vi "Get JSON Data.vi"(7 "Panel Origin":T1, 8 "error in (no error)":errorcluster, 9 "Force Get All Data":bool, 10 "VI Reference":refnum<vi>, 11 "Boolean In":refnum<class "Boolean.lvclass">) -> (0 "error out":errorcluster, 2 "JSON string":string, 3 "Boolean Out":refnum<class "Boolean.lvclass">)   [LabVIEW 2015, in "Front Panel Publisher.lvlib" / "Boolean.lvclass"]
uses:
  Boolean.lvclass
  <vilib>/Utility/miscctls.llb/LVPointTypeDef.ctl
  Text_class/Text.lvclass
  Control_class/Control.lvclass
  Object_class/Object.lvclass
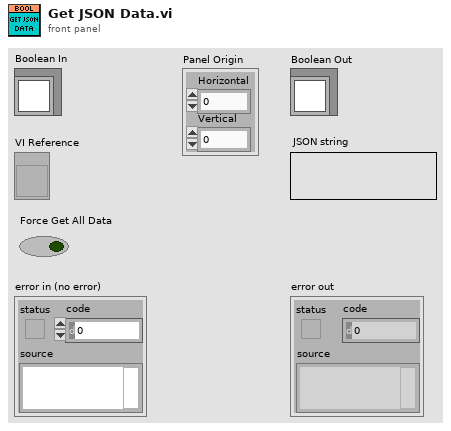
[diagram p1: front panel]
types:
  T1 = typedef "LVPointTypeDef.ctl" = cluster{"Horizontal":i16, "Vertical":i16}
  T2 = typedef "Front Panel Publisher.lvlib/Object.lvclass/Attributes.ctl" = cluster{"UID":i32, "Type":string, "Coordinates":T3, "Reference":refnum<vi>}
  T3 = typedef "Front Panel Publisher.lvlib/Object.lvclass/Coordinates.ctl" = cluster{"Left":i32, "Top":i32, "Height":u32, "Width":u32}
  T4 = typedef "Front Panel Publisher.lvlib/Control.lvclass/Attributes.ctl" = cluster{"Description":string, "Indicator":bool, "Default Value":variant, "Control Index":i32, "Label":refnum<class "Text.lvclass">, "Caption":refnum<class "Text.lvclass">, "Image b64":string, "Use Picture":bool, "Value Only":bool}
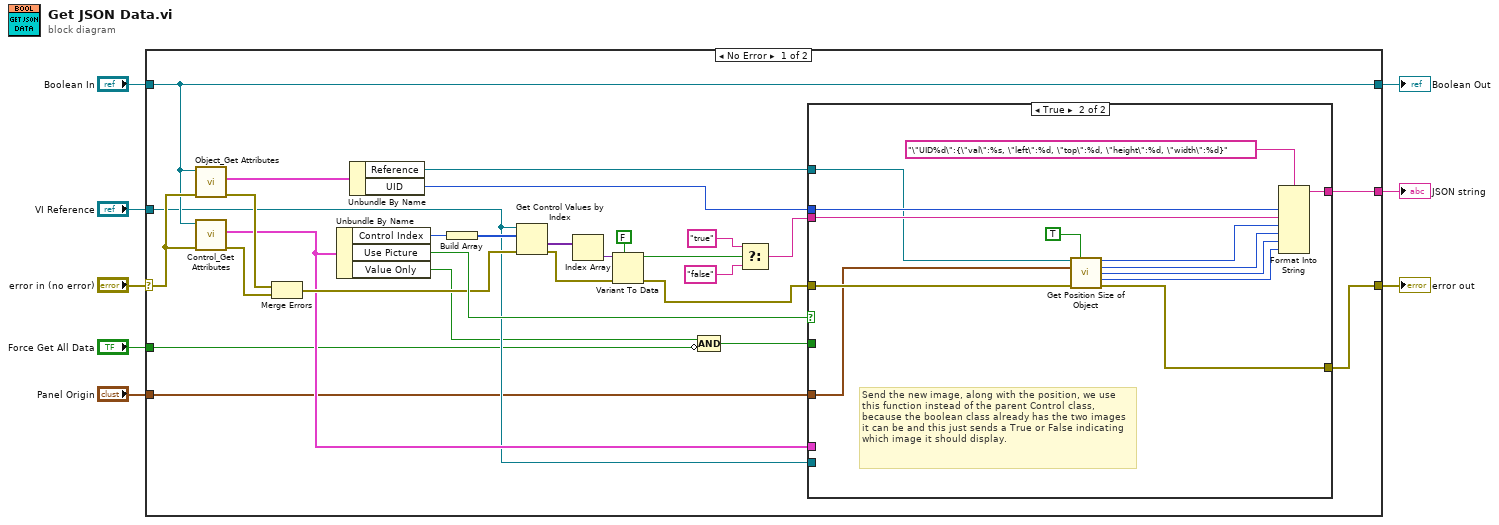
[diagram p0: block diagram]
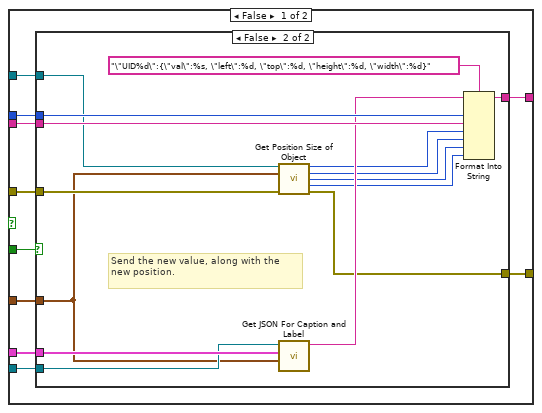
[diagram p2: hidden frame]
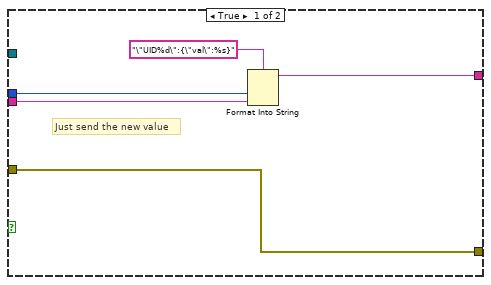
[diagram p3: hidden frame]
diagram:
  n1 = case shown="No Error" "error in (no error)" {
    selector: "error in (no error)" -> [w34 w81]
    tunnel: [w35 w81] -> w7
    tunnel: [w31 w80] -> w5
    tunnel: "Boolean In" -> [w31 w80]
    tunnel: "VI Reference" -> [w13 _]
    tunnel: [w32 _] -> w3
    tunnel: "Force Get All Data" -> [w11 _]
    tunnel: "Panel Origin" -> [w9 _]
    frame No Error {
      n2 = call "Object_Get Attributes.vi"("error in (no error)"=w34, "Object In"=w31) -> ("error out"=w15:errorcluster, "Data"=w30:T2)  [unwired: 6 in, 2 out]
      n3 = call "Control_Get Attributes.vi"("error in (no error)"=w34, "Control In"=w31) -> ("error out"=w36:errorcluster, "Data"=w14:T4)  [unwired: 6 in, 2 out]
      n4 = Merge Errors(w15, w36) -> (w16:errorcluster)
      n5 = Unbundle By Name(w14) -> ("Control Index"=w33:i32, "Use Picture"=w18:bool, "Value Only"=w12:bool)
      n6 = Unbundle By Name(w30) -> ("Reference"=w17:refnum<vi>, "UID"=w29:i32)
      n7 = Build Array(w33) -> (w26:i32[])
      n8 = Get Control Values by Index(0:w13, 1:w26, 3:w16) -> (10:w25:variant[], 11:w28:errorcluster)
      n9 = Index Array(array=w25) -> (element=w24:variant)  [unwired: 1 in]
      n10 = Variant To Data(error in=w28, type=FALSE, Variant=w24) -> (data=w22:bool, error out=w27:errorcluster)
      n11 = Compound Arithmetic op=AND(w12, invert w11) -> (w10:bool)
      n12 = Select(t="true", s=w22, f="false") -> (s? t:f=w19:string)
      n13 = case shown="True" w18 {
        tunnel: [w41 w69] -> w35
        tunnel: [w46 w76] -> w32
        tunnel: w29 -> [w45 w78]
        tunnel: w27 -> [w42 w74]
        tunnel: w19 -> [w44 w77]
        tunnel: w17 -> [w40 w75]
        tunnel: w10 -> [w43 _]
        tunnel: w14 -> [w39 _]
        tunnel: w13 -> [w38 _]
        tunnel: w9 -> [w37 w67]
        frame False {
          n14 = case shown="False" w43 {
            tunnel: [w51 w66] -> w46
            tunnel: w45 -> [w50 w65]
            tunnel: w44 -> [w48 w63]
            tunnel: w42 -> [w47 w54]
            tunnel: [w47 w53] -> w41
            tunnel: w40 -> [_ w59]
            tunnel: w39 -> [_ w62]
            tunnel: w38 -> [_ w61]
            tunnel: w37 -> [_ w52]
            frame True {
              # "Just send the new value"
              n15 = Format Into String(format string="\"UID%d\":{\"val\":%s}", w50, w48) -> (resulting string=w51:string)  [unwired: 2 in, 1 out]
            }
            frame False {
              # "Send the new value, along with the new position."
              n16 = call "Get Position Size of Object.vi"("GObject in"=w59, "Panel Origin"=w52, "error in (no error)"=w54) -> ("Left"=w58:i32, "Top"=w57:i32, "Height"=w56:u32, "Width"=w55:u32, "error out"=w53:errorcluster)  [unwired: 8 in]
              n17 = call "Get JSON For Caption and Label.vi"("Panel Origin"=w52, "Data"=w62, "VI in"=w61) -> ("JSON"=w60:string)  [unwired: 7 in, 1 out]
              n18 = Format Into String(format string="\"UID%d\":{\"val\":%s, \"left\":%d, \"top\":%d, \"height\":%d, \"width\":%d}", initial string=w60, w65, w63, w58, w57, w56, w55) -> (resulting string=w66:string)  [unwired: 1 in, 1 out]
            }
          }
        }
        frame True {
          # "Send the new image, along with the position, we use this function instead of the parent Control class, because the boolean class already has the two images it can be and this just sends a True or False indicating which image it should display."
          n19 = call "Get Position Size of Object.vi"("GObject in"=w75, "Use Total Rect"=TRUE, "Panel Origin"=w67, "error in (no error)"=w74) -> ("Left"=w73:i32, "Top"=w72:i32, "Height"=w71:u32, "Width"=w70:u32, "error out"=w69:errorcluster)  [unwired: 7 in]
          n20 = Format Into String(format string="\"UID%d\":{\"val\":%s, \"left\":%d, \"top\":%d, \"height\":%d, \"width\":%d}", w78, w77, w73, w72, w71, w70) -> (resulting string=w76:string)  [unwired: 2 in, 1 out]
        }
      }
    }
    frame Error {
    }
  }
  "error out" <- w7
  "Boolean Out" <- w5
  "JSON string" <- w3
